vi "Auton Maxtime.vi"(10 "MaxTime":dbl, 11 "Reset?":bool) -> (1 "Finished?":bool)   [LabVIEW 2017]
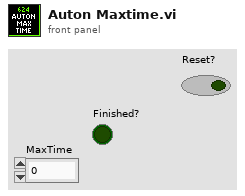
[diagram p1: front panel]
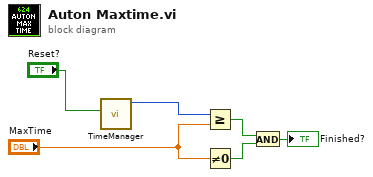
[diagram p0: block diagram]
diagram:
  n1 = call "TimeManager.vi"("Reset?"="Reset?") -> ("Time Since Reset"=w3:u32)  [unwired: 9 in, 1 out]
  n2 = Greater Or Equal?(x=w3, y="MaxTime") -> (x >= y?=w6:bool)
  n3 = Not Equal To 0?(x="MaxTime") -> (x != 0?=w5:bool)
  n4 = And(x=w6, y=w5) -> (x .and. y?=→"Finished?":bool)
